vi "FindMaxnIndex.vi"(8 "error in (no error)":errorcluster) -> (0 "error out":errorcluster, 1 "Numeric":i32, 3 "String":string)   [LabVIEW 2020]
uses:
  <vilib>/Utility/file.llb/Read Delimited Spreadsheet (string).vi
panel:
  out "number":i32[][](array[numeric])
  out "all rows":string[][](array[string])
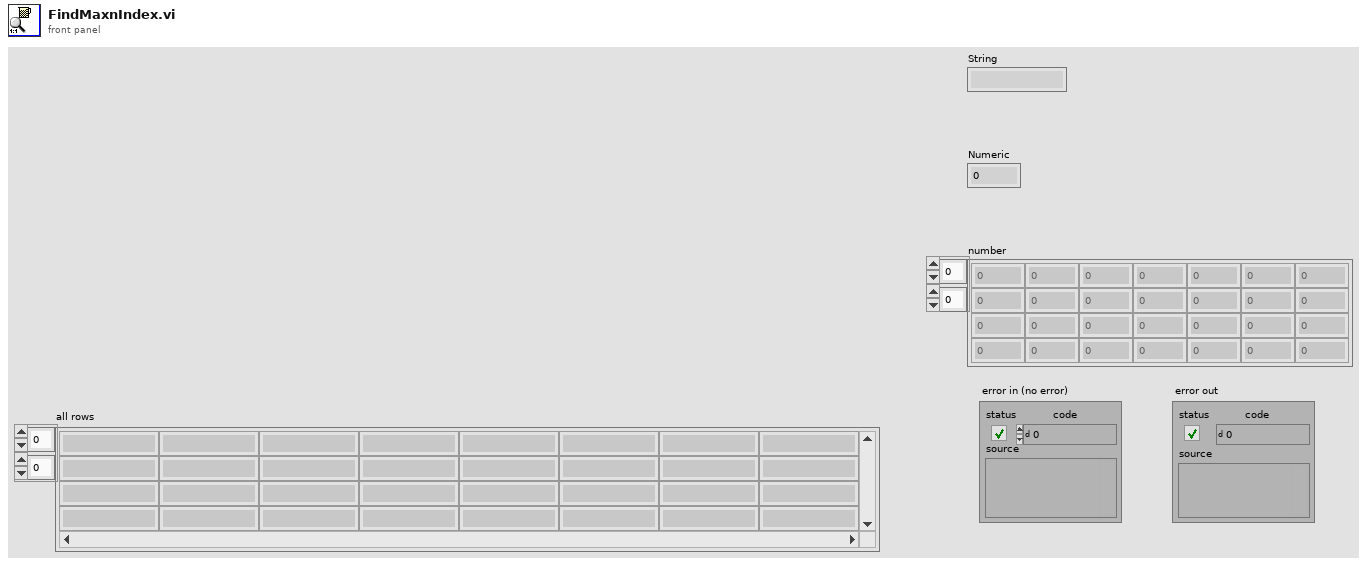
[diagram p1: front panel]
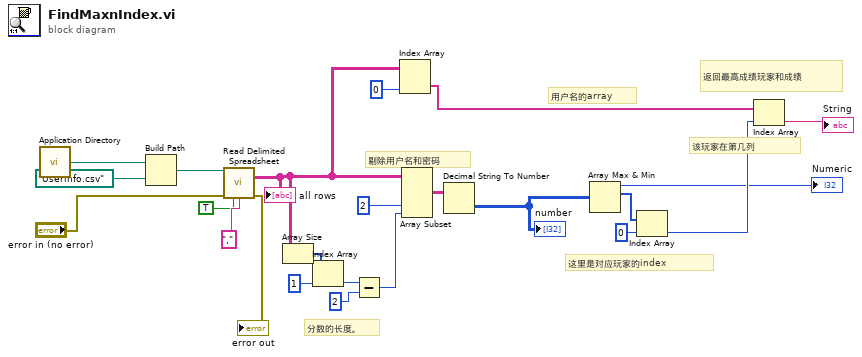
[diagram p0: block diagram]
diagram:
  # "分数的长度。"
  # "用户名的array"
  # "该玩家在第几列"
  # "返回最高成绩玩家和成绩"
  # "剔除用户名和密码"
  # "这里是对应玩家的index"
  n1 = call <vilib>:"Application Directory.vi"() -> ("Application Directory"=w7:path)
  n2 = Build Path(base path=w7, name or relative path=path "Userinfo.csv") -> (appended path=w3:path)
  n3 = call-poly <vilib>:"Read Delimited Spreadsheet.vi"("file path (dialog if empty)"=w3, "error in (no error)"="error in (no error)", "transpose? (F)"=TRUE, "delimiter (\\t)"="," ("delimiter (\\t)")) -> ("all rows"=w19:string[][], "error out"=→"error out":errorcluster)  [unwired: 6 in, 4 out]
  "all rows" <- w19
  n4 = Array Size(array=w19) -> (size(s)=w9:i32[])
  n5 = Index Array(array=w9, index=1) -> (element=w11:i32)
  n6 = Subtract(x=w11, y=2 ("index")) -> (x-y=w13:i32)
  n7 = Index Array(array=w19, index (col)=0 ("index (row)")) -> (element=w22:string[])  [unwired: 1 in]
  n8 = Array Subset(array=w19, index (col)=2 ("index"), length (col)=w13) -> (w14:string[][])  [unwired: 2 in]
  n9 = Decimal String To Number(string=w14) -> (number=w16:i32[][])  [unwired: 2 in, 1 out]
  "number" <- w16
  n10 = Array Max & Min(array=w16) -> (max value=→"Numeric":i32, max index (indices)=w18:i32[])  [unwired: 2 out]
  n11 = Index Array(array=w18, index=0) -> (element=w21:i32)
  n12 = Index Array(array=w22, index=w21) -> (element=→"String":string)
